vi "CCD_Exposure_2-D.vi"(7 "CCD GPIB Address":u16=1, 8 "error in":errorcluster, 10 "Shutter Enabled":bool=TRUE, 11 "Exposuretime (s)":dbl=0.5 format="%.2f") -> (0 "Error Out":errorcluster, 1 "#PixelOverflow":u32, 2 "PixelOverflow":bool, 3 "The Data":i32[][](array[numeric]), 4 "SD":i32=1024, 5 "1-D data":i32[](graph)=[177496, 177237, 176545, 175663, 175741, 175858, 175364, 175697, 175129, 174991, 175361, 175049, 173976, 174267, 174715, 174635, 174464, 174415, 174713, 174154, 174258, 174337, 173766, 174440, 174836, 174872, 175484, 175380, 175517, 175102, 176092, 175373, 177070, 176721, 176679, 176652, 176571, 177207, 176449, 176451, 176423, 175916, 176475, 176612, 176252, 176325, 176549, 176615, 176346, 176479, 175031, 175855, 175811, 175987, 175754, 176075, 175744, 176016, 176357, 176668, 175778, 176616, 176413, 176166, 176151, 176171, 176217, 176658, 176512, 175690, 176874, 176617, 176661, 176440, 176822, 176737, 176660, 176897, 177128, 176173, 176955, 177131, 176857, 177057, 177128, 177374, 177408, 177629, 176564, 177537, 178203, 177779, 177922, 178109, 178176, 177927, 177938, 178018, 178044, 178507, 178492, 178457, 178751, 178462, 179124, 178828, 178898, 178567, 179197, 179313, 179250, 178875, 179058, 179277, 179500, 179982, 179462, 179335, 179263, 179484, 179481, 179479, 179610, 179444, 179554, 179661, 178821, 179552, 179705, 179488, 179515, 179423, 179453, 179461, 179755, 179369, 179414, 179479, 179807, 179976, 179789, 179795, 179568, 179889, 179778, 178767, 179542, 179786, 179938, 179612, 179142, 179106, 179581, 179567, 178634, 178623, 179068, 178940, 178900, 178928, 179101, 178915, 178740, 178763, 177499, 178666, 178321, 178221, 178009, 178053, 177909, 177925, 177857, 177602, 177533, 177626, 177249, 177582, 177192, 176946, 177060, 176820, 176649, 175734, 176509, 176182, 176157, 176331, 176091, 176038, 175744, 176229, 175506, 175197, 175508, 175642, 175167, 175458, 175353, 175323, 175173, 175444, 174506, 175316, 175313, 175117, 174765, 174432, 175002, 174688, 174440, 173961, 174115, 174147, 174093, 173735, 173903, 173716, 173765, 173610, 173748, 173011, 173245, 173618, 173124, 173369, 173061, 173038, 172885, 172760, 172514, 172554, 173031, 173023, 172516, 172523, 172672, 172471, 172237, 172188, 171433, 171984, 171753, 171872, 171783, 171471, 171189, 171110, 171274, 170575, 171120, 171106, 171110, 170929, 171173, 170662, 170816, 170628, 170624, 170225, 170081, 170283, 170029, 169998, 169688, 169824, 169406, 169878, 169063, 169720, 169510, 169519, 169860, 169714, 169518, 169643, 169456, 169521, 168869, 169560, 168783, 168901, 168990, 169036, 168442, 168777, 168687, 168072, 168399, 168649, 168267, 168269, 168356, 168516, 168271, 168527, 167836, 167485, 167850, 167521, 167426, 167557, 167423, 167443, 167534, 167009, 166530, 167863, 167026, 166940, 167186, 166745, 166891, 166955, 166869, 167115, 165754, 166348, 166107, 166618, 166316, 166267, 166555, 166327, 166013, 165723, 166506, 166349, 165892, 166071, 166190, 165856, 165930, 165701, 165506, 164608, 165119, 165024, 165449, 165200, 165259, 165019, 165349, 164958, 164096, 165006, 164981, 164335, 164861, 164810, 164423, 164483, 164340, 164250, 163491, 164245, 164320, 163963, 163883, 163507, 163916, 164060, 164046, 162766, 163198, 163532, 163551, 163543, 162990, 163030, 163314, 163224, 162808, 162701, 162758, 162941, 163168, 162957, 163135, 162477, 162607, 162991, 161590, 162713, 162532, 162527, 162445, 162391, 162501, 162180, 162584, 162352, 162069, 162010, 161850, 162592, 162134, 161802, 161889, 161835, 162271, 161372, 161806, 161901, 161746, 161668, 161955, 161987, 161665, 161955, 161624, 161234, 161128, 161451, 161255, 161395, 161342, 161345, 161407, 161028, 160195, 161186, 160747, 160842, 160504, 160787, 160732, 160423, 160488, 160268, 159891, 159897, 160079, 160098, 160144, 159838, 160097, 160087, 159870, 159061, 159506, 159511, 159803, 159529, 159439, 159512, 158853, 159324, 158534, 159173, 159332, 158882, 159051, 158572, 158514, 158829, 158706, 158748, 157912, 158607, 158090, 158227, 158152, 158030, 158266, 158548, 158016, 157962, 158035, 157954, 157812, 157606, 157874, 157821, 157764, 157655, 157657, 156469, 156933, 156940, 156737, 156720, 156676, 156742, 156663, 156501, 156267, 156025, 156139, 156305, 155684, 155848, 155778, 156013, 155699, 155868, 155073, 155035, 154988, 155147, 155006, 154801, 154951, 154756, 154369, 154043, 154641, 154227, 154445, 154230, 154204, 154021, 153772, 153607, 154029, 152755, 153333, 153458, 153185, 152741, 152835, 152962, 152667, 152345, 151613, 152074, 152206, 152113, 151817, 151704, 151180, 151839, 151412, 150982, 150417, 151000, 150816, 150477, 150540, 150350, 150468, 150158, 149893, 149892, 149892, 149939, 149467, 149632, 149759, 149220, 148925, 149026, 148528, 147863, 148334, 148442, 148328, 147973, 148089, 148183, 148195, 147150, 146769, 147095, 147236, 146926, 146726, 146613, 146268, 146185, 145926, 146010, 144893, 145439, 145063, 145105, 144597, 144535, 143936, 143844, 143722, 142725, 142943, 143042, 142449, 142272, 142469, 141769, 141972, 141248, 141044, 140226, 140827, 140698, 140582, 139873, 140115, 139849, 139848, 139546, 138440, 138703, 138359, 138382, 138330, 137878, 137475, 137443, 137045, 136996, 136153, 136373, 136062, 135957, 135597, 135569, 135341, 135358, 135207, 133688, 134368, 133832, 134099, 133500, 133809, 133295, 132918, 132596, 131737, 131215, 131598, 130920, 131159, 130586, 129849, 130121, 129509, 129389, 128346, 128603, 127886, 127724, 127466, 127149, 126899, 126396, 126106, 125250, 125243, 125186, 124756, 124152, 124208, 123733, 123689, 123302, 122709, 121638, 122192, 121550, 121617, 121037, 121065, 121206, 120503, 120291, 120082, 119444, 119479, 119102, 119126, 118821, 119007, 119014, 118790, 118557, 117857, 118423, 117958, 118209, 118033, 117577, 117864, 117940, 117602, 117323, 117173, 117415, 117204, 117219, 116831, 117214, 116727, 116894, 116543, 116291, 116423, 116250, 116254, 115966, 115960, 116156, 115985, 115893, 115539, 115492, 115586, 115303, 115517, 115319, 115197, 115309, 114934, 115043, 114792, 114926, 114745, 114650, 114608, 114556, 114530, 114548, 114068, 113966, 114303, 114062, 114250, 113447, 113715, 113923, 113602, 113622, 113621, 113042, 113452, 113341, 113201, 113118, 113203, 112990, 112896, 112779, 112551, 112388, 112593, 112630, 112401, 112398, 112425, 112142, 112350, 112104, 111345, 111918, 111650, 111627, 111487, 111664, 111526, 111384, 111199, 111222, 111185, 111051, 111127, 110794, 110856, 111102, 110991, 110891, 110806, 110318, 110703, 110754, 110560, 110283, 110215, 110234, 110522, 110338, 109585, 110017, 109557, 109843, 109787, 109970, 109426, 109645, 109169, 109373, 108726, 109269, 109089, 109002, 109200, 109471, 108942, 109150, 108845, 108649, 108633, 108861, 108788, 108644, 108488, 108826, 108492, 108466, 108611, 107787, 107908, 108145, 108047, 107821, 107704, 107751, 107942, 107756, 107019, 107515, 107226, 107147, 107147, 107373, 107606, 106987, 107275, 106973, 106570, 106853, 107103, 106538, 106818, 106677, 106780, 106598, 106569, 106075, 106391, 106148, 106190, 106330, 106036, 106176, 106260, 106130, 105583, 105341, 105443, 105751, 105576, 105607, 105404, 105402, 105428, 105391, 104782, 105311, 105399, 105205, 104839, 105129, 105010, 104872, 104917, 104547, 104139, 104521, 104271, 104632, 104550, 104222, 104145, 104298, 104354, 103669, 104110, 103604, 104021, 103788, 103749, 103773, 103624, 103645, 103361, 103629, 103258, 103289, 103247, 103211, 103330, 103247, 103436, 103179, 102579, 102963, 102898, 102864, 102648, 102776, 102586, 102631, 102257, 102254, 102088, 102615, 102228, 102414, 102386, 102025, 101999, 101883, 101846, 101309, 101626, 101609, 101613, 101571, 101653, 101255, 101350, 101514, 100925, 100796, 101115, 100842, 101202, 100630, 100907, 100811, 100773, 100654, 100153, 100255, 100664, 100226, 100257, 100301, 99998, 100192, 99883, 99797, 99144, 99679, 99809, 99363, 99594, 99253, 99180, 99343, 99103, 98304, 99091, 98839, 98869, 98550, 98599, 98609, 98348, 98588, 98238, 97988, 98192, 97809, 97831, 97989, 97745, 97967, 97680, 97445, 96931, 97422, 97486, 97364, 97247, 97010, 96943, 96835, 96708, 96620, 96687, 96317, 96392, 96030, 96281, 95988, 96006, 95720, 96009, 95349, 95599, 95334, 95322, 95474, 95161, 95122, 94994, 95082, 94621, 94507, 94795, 94877, 94686, 94852, 94530, 94409, 94757, 94791, 94046, 94197, 94237, 94125, 93995, 94019, 94245, 94207, 94286, 93544, 93928, 93947, 93713, 94034, 93985, 91259], 6 "Setup String":string="ldb,1,0,u,0,180,30,b,1,76;sdu,0,1024,1024;cl0;omrt;sron;she;ex0.2")   [LabVIEW 2020]
doc: "Get the 2-D CCD data. The CCD GPIB address is more or less fixed.\nThe setup string uses global variable."
uses:
  Globals and TypeDefs/Type Definitions.llb/3 way Status.ctl
  Globals and TypeDefs/gStatus.vi
  Globals and TypeDefs/gDetector.vi
panel:
  out "SRQ":bool[](array[boolean])
  out "Trailing Byte":bool[](array[boolean])
  out "Trailing Byte Str":string
  out "#Mismatched":u32
  out "Bytes for Readout":i32
  out "Read String length":i32
  out "#Read Error":u32
  out "#SRQ Error":u32
  out "#Shots":u32
  out "Intensity Graph":i32[][](graph)
  out "Current State":T1(ring)=enum."Send Command"
  out "Data Dimensions":i32[](array[numeric])=[1024, 30]
  out "read":bool[](array[boolean])=[FALSE, FALSE, FALSE, FALSE, FALSE, FALSE, FALSE, FALSE, TRUE, FALSE, FALSE, FALSE, FALSE, TRUE, FALSE, FALSE]
  out "TS":bool[](array[boolean])
  out "ST":bool[](array[boolean])=[FALSE, FALSE, FALSE, FALSE, FALSE, FALSE, FALSE, FALSE, TRUE, FALSE, FALSE, FALSE, FALSE, FALSE, FALSE, FALSE]
  out "SRQ poll response":i16=65
  out "InitialArray Length":i32=30720
  out "LD":i32=30
  # "Acc overflow"
  # "FIFO overflow"
  # "Exp halted by user"
  # "Status Byte:\n[0]: Dev.Clear State  \n[1]: Dev.Trig.State    \n[2]: Listener Active   \n[3]: Talker Active      \n[4]: Attn. Asserted    \n[5]: CIC                      \n[6]: Remote State       \n[7]: Lockout State      \n[8]: Oper.Complete\n[9]:   ---\n[10]: ---\n[11]: ---\n[12]: SRQ det.whl CIC\n[13]: EOI or EOS det.\n[14]: Timeout\n[15]: Error detected"
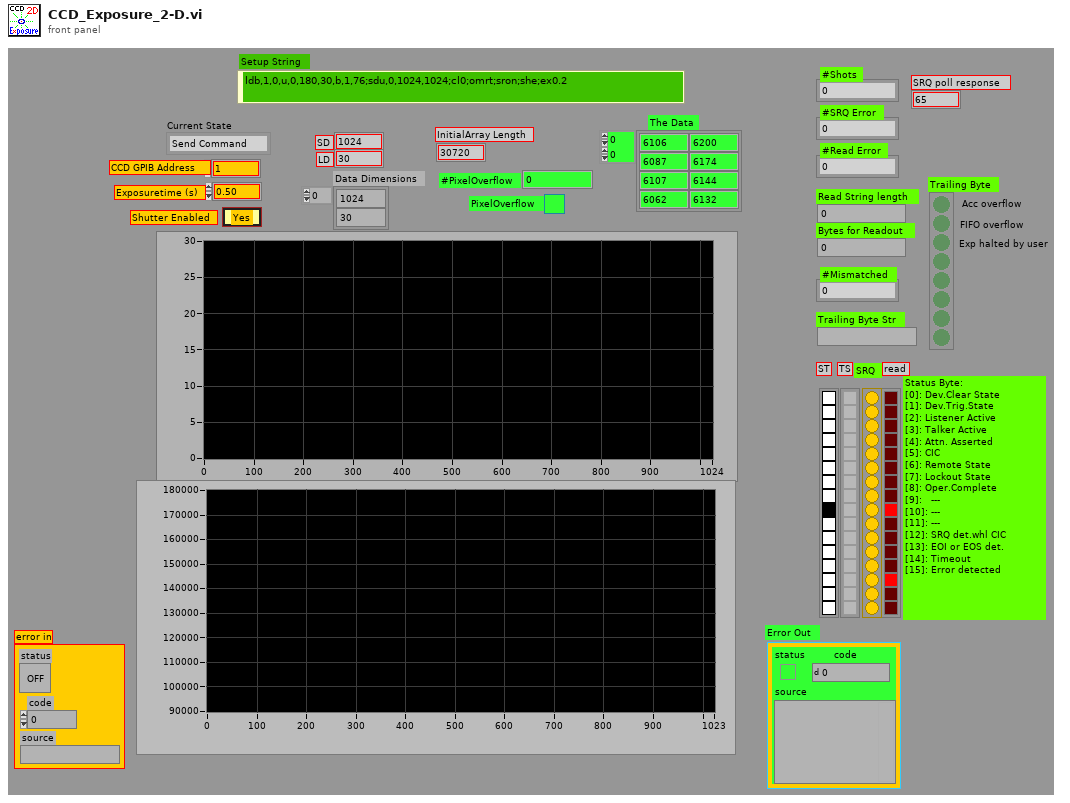
[diagram p1: front panel]
types:
  T1 = enum16{"__Quit__", "Send Command", "Wait", "Check SRQ", "Receive Data"}
  T2 = typedef "3 way Status.ctl" = u8
  T3 = enum16{"__Quit__", "Send Command", "Wait", "Check SRQ", "Receive Data", "Process Data"}
  T4 = enum16{"--Quit--", "Init GPIB", "Poll GPIB", "Wait for SRQ", "Clear CCD Parameters", "New CCD Parameters", "Check CCD Command Error"}
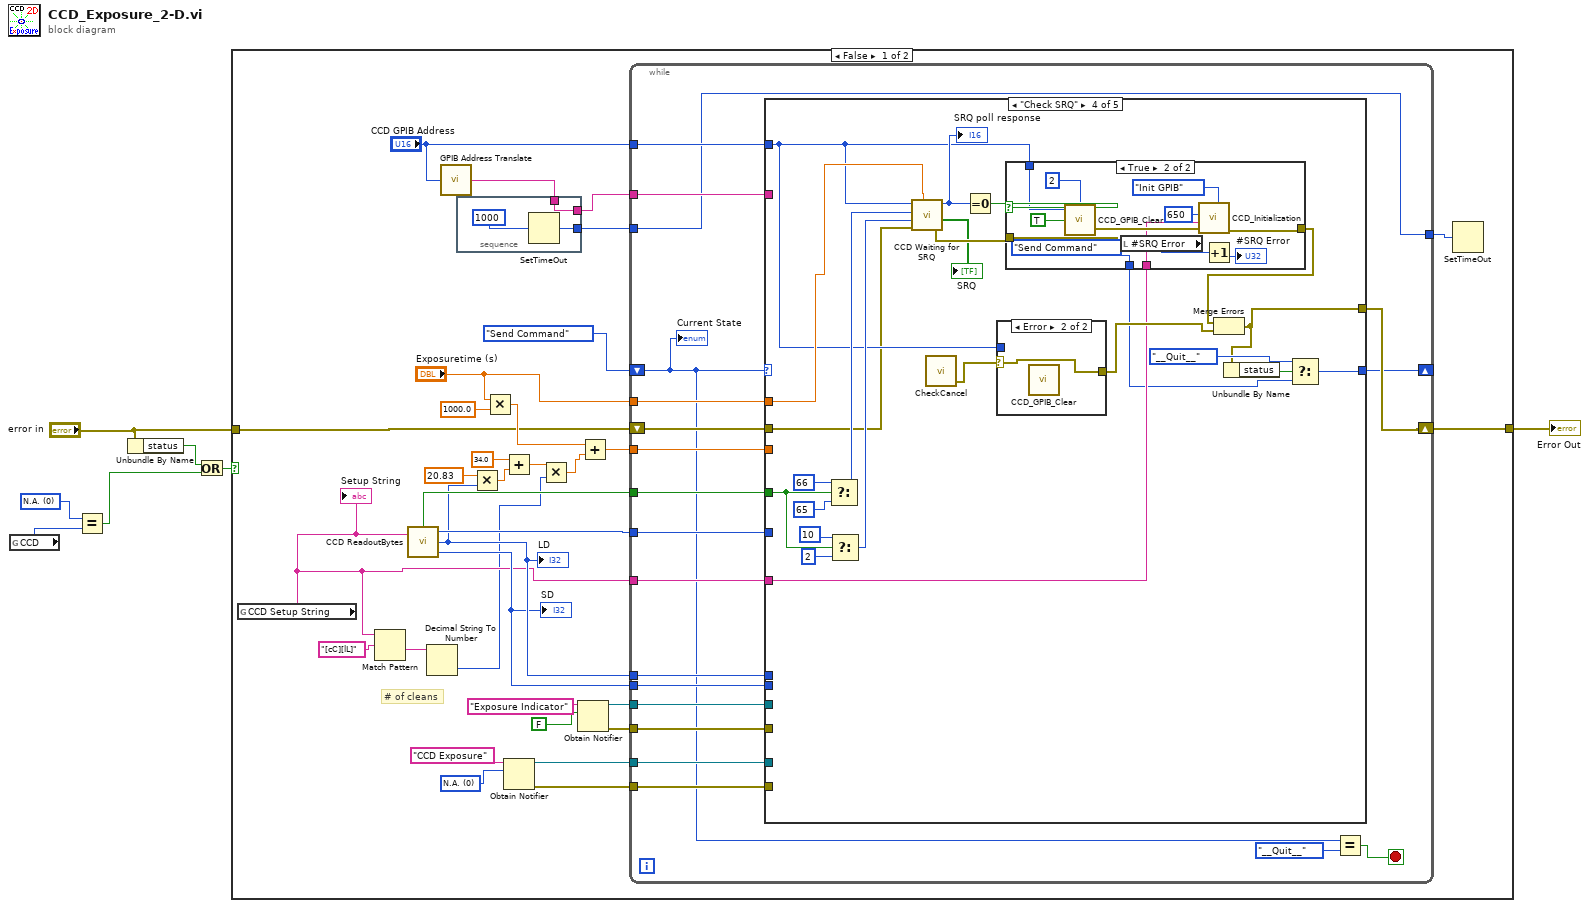
[diagram p0: block diagram]
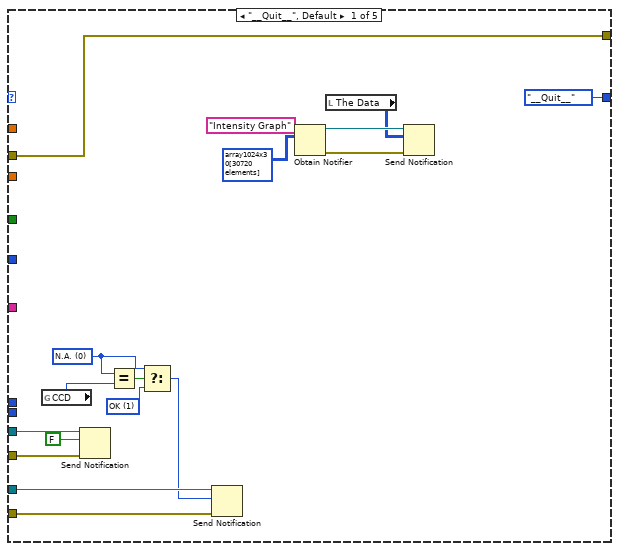
[diagram p2: hidden frame]
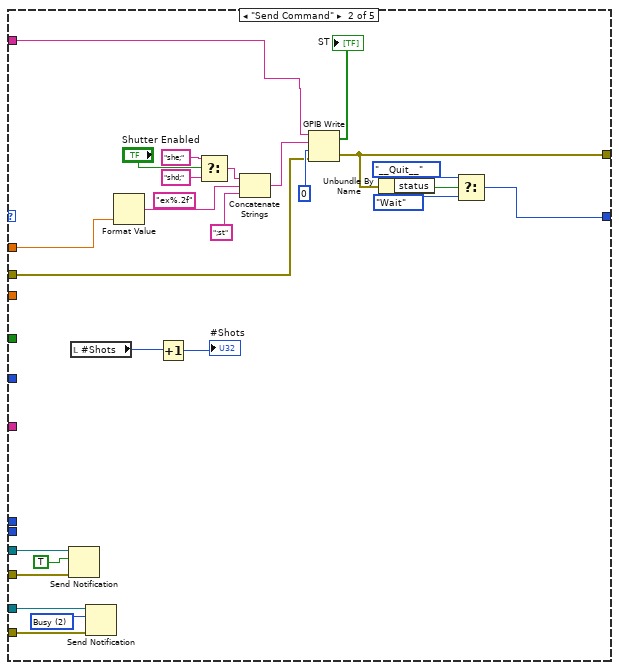
[diagram p3: hidden frame]
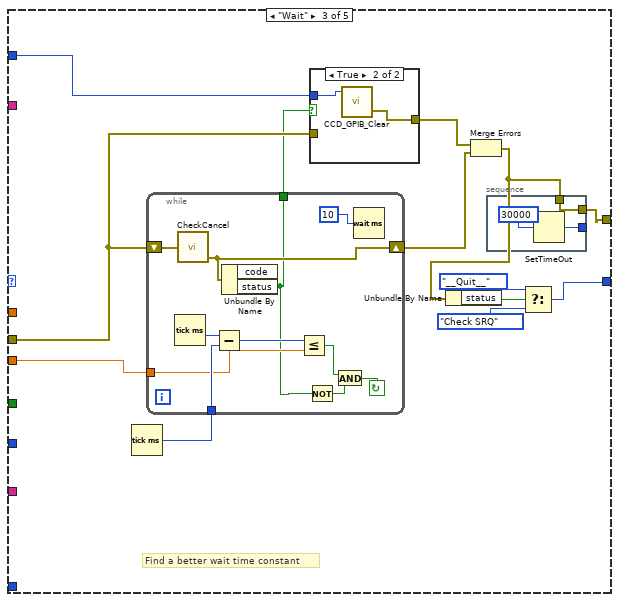
[diagram p4: hidden frame]
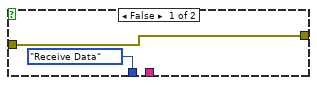
[diagram p6: hidden frame]
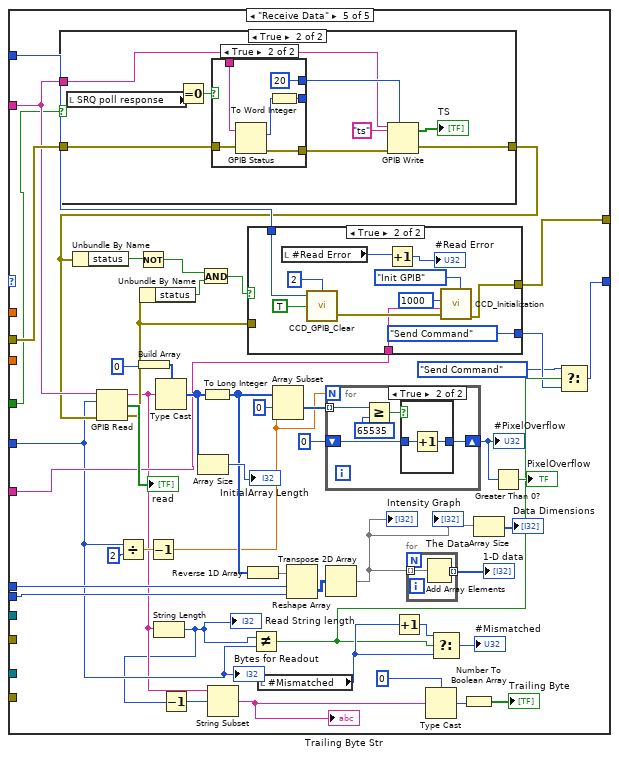
[diagram p8: hidden frame]
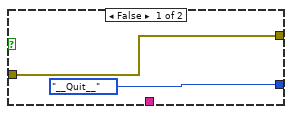
[diagram p9: hidden frame]
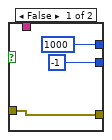
[diagram p11: hidden frame]
diagram:
  w5 = T2 0 items=["N.A.", "OK", "Busy", "Done"] ("y")
  n1 = global read "gStatus.vi" "CCD"() -> (w6:T2)
  n2 = Equal?(x=w5, y=w6) -> (x = y?=w3:bool)
  n3 = Unbundle By Name("error in") -> ("status"=w2:bool)
  n4 = Or(x=w2, y=w3) -> (x .or. y?=w4:bool)
  n5 = case shown="False" w4 {
    tunnel: [w27 w265] -> w7
    tunnel: "error in" -> [w25 w265]
    frame False {
      w14 = T2 0 items=["N.A.", "OK", "Busy", "Done"] ("Saving")
      # "# of cleans"
      n6 = global read "gDetector.vi" "CCD Setup String"() -> (w20:string)
      "Setup String" <- w20
      n7 = Match Pattern(string=w20, regular expression="[cC][lL]") -> (after substring=w21:string)  [unwired: 1 in, 3 out]
      n8 = call "CCD ReadoutBytes.vi"("CCD Setup String"=w20) -> ("RM(T) or RT(F) mode"=w37:bool, "Bytes for Readout"=w38:i32, "LD Bytes"=w29:i32, "SD Bytes"=w28:i32)  [unwired: 1 in]
      "SD" <- w28
      "LD" <- w29
      n9 = Decimal String To Number(string=w21) -> (number=w18:i32)  [unwired: 2 in, 1 out]
      n10 = call "GPIB Address Translate.vi"("GPIB Address"="CCD GPIB Address") -> ("GPIB Address String"=w40:string)
      n11 = stacked-sequence {
        tunnel: [w42] -> w39
        tunnel: w40 -> [w42]
        tunnel: [w41] -> w24
        frame #0 {
          n12 = SetTimeOut(1:1000) -> (0:w41:i32)
        }
      }
      n13 = Multiply(x=20.83, y=w29) -> (x*y=w35:dbl)
      n14 = Multiply(x="Exposuretime (s)", y=1000.0) -> (x*y=w31:dbl)
      n15 = Add(x=34.0, y=w35) -> (x+y=w19:dbl)
      n16 = Obtain Notifier(name (unnamed)="CCD Exposure", notification data type=w14) -> (notifier out=w13:refnum<notifier>, error out=w12:errorcluster)  [unwired: 2 in, 1 out]
      n17 = Multiply(x=w19, y=w18) -> (x*y=w17:dbl)
      n18 = Obtain Notifier(name (unnamed)="Exposure Indicator", notification data type=FALSE ("SaveData?")) -> (notifier out=w9:refnum<notifier>, error out=w8:errorcluster)  [unwired: 2 in, 1 out]
      n19 = Add(x=w31, y=w17) -> (x+y=w16:dbl)
      n20 = while {
        shift-right: [w59] -> _
        shift-left: T1."Send Command" ("Starting Mode") -> [w44]
        tunnel: w39 -> [w63]
        shift-right: [w61] -> w27
        shift-left: w25 -> [w62]
        tunnel: w38 -> [w56]
        tunnel: w37 -> [w57]
        tunnel: "Exposuretime (s)" -> [w60]
        tunnel: "CCD GPIB Address" -> [w58]
        tunnel: w29 -> [w55]
        tunnel: w28 -> [w54]
        tunnel: w20 -> [w51]
        tunnel: w24 -> [w50]
        tunnel: [w50] -> w23
        tunnel: w16 -> [w49]
        tunnel: w13 -> [w48]
        tunnel: w12 -> [w47]
        tunnel: w9 -> [w46]
        tunnel: w8 -> [w45]
        stop <- w53 stop-if-true
        n21 = case shown="\"Check SRQ\"" w44 {
          tunnel: w63 -> [_ w96 _ _ w204]
          tunnel: w62 -> [w77 w95 w115 w138 w222]
          tunnel: [w77 w93 w108 w154 w191] -> w61
          tunnel: w60 -> [_ w94 _ w147 _]
          tunnel: [T3."__Quit__" w89 w111 w153 w177] -> w59
          tunnel: w58 -> [_ _ w118 w140 w198]
          tunnel: w57 -> [_ _ _ w151 w199]
          tunnel: w56 -> [_ _ _ _ w189]
          tunnel: w55 -> [_ _ _ _ w203]
          tunnel: w54 -> [_ _ _ _ w202]
          tunnel: w51 -> [_ _ _ w142 w190]
          tunnel: w49 -> [_ _ w110 _ _]
          tunnel: w48 -> [w79 w86 _ _ _]
          tunnel: w47 -> [w78 w85 _ _ _]
          tunnel: w46 -> [w71 w83 _ _ _]
          tunnel: w45 -> [w70 w82 _ _ _]
          frame "__Quit__", Default {
            w73 = T2 1 items=["N.A.", "OK", "Busy", "Done"] ("f")
            w74 = T2 0 items=["N.A.", "OK", "Busy", "Done"] ("y")
            n22 = global read "gStatus.vi" "CCD"() -> (w75:T2)
            n23 = Send Notification(notification=FALSE, notifier=w71, error in (no error)=w70) -> ()  [unwired: 2 out]
            n24 = Equal?(x=w74, y=w75) -> (x = y?=w76:bool)
            n25 = Select(t=w74, s=w76, f=w73) -> (s? t:f=w72:T2)
            n26 = Send Notification(notification=w72, notifier=w79, error in (no error)=w78) -> ()  [unwired: 2 out]
            n27 = Obtain Notifier(name (unnamed)="Intensity Graph", notification data type=i32[][] array1024x30[30720 elements] ("Intensity Graph")) -> (notifier out=w66:refnum<notifier>, error out=w65:errorcluster)  [unwired: 2 in, 1 out]
            n28 = local read "The Data"() -> (w64:i32[][])
            n29 = Send Notification(notification=w64, notifier=w66, error in (no error)=w65) -> ()  [unwired: 2 out]
          }
          frame "Send Command" {
            w84 = T2 2 items=["N.A.", "OK", "Busy", "Done"] ("notification")
            n30 = Send Notification(notification=TRUE, notifier=w83, error in (no error)=w82) -> ()  [unwired: 2 out]
            n31 = local read "#Shots"() -> (w87:u32)
            n32 = Send Notification(notification=w84, notifier=w86, error in (no error)=w85) -> ()  [unwired: 2 out]
            n33 = Format Value(format string="ex%.2f", value (0)=w94) -> (output string=w104:string)  [unwired: 1 in]
            n34 = Increment(x=w87) -> (x+1=→"#Shots":u32)
            n35 = Select(t="she;", s="Shutter Enabled", f="shd;") -> (s? t:f=w103:string)
            n36 = Concatenate Strings(w103, w104, ";st") -> (w105:string)
            n37 = GPIB Write(0:w96, 1:w105, 2:i16 0 ("mode (0)"), 3:w95) -> (5:→"ST":bool[], 6:w93:errorcluster)  [unwired: 1 in]
            n38 = Unbundle By Name(w93) -> ("status"=w92:bool)
            n39 = Select(t=T3."__Quit__", s=w92, f=T3."Wait" ("Starting Mode")) -> (s? t:f=w89:T3)
          }
          frame "Wait" {
            # "Find a better wait time constant"
            n40 = Tick Count (ms)() -> (millisecond timer value=w119:u32)
            n41 = while {
              tunnel: w110 -> [w133]
              tunnel: w119 -> [w135]
              shift-right: [w127] -> w116
              shift-left: w115 -> [w128]
              tunnel: [w126] -> w109
              stop <- w130 continue-if-true
              n42 = Tick Count (ms)() -> (millisecond timer value=w136:u32)
              n43 = call "CheckCancel.vi"("error in (no error)"=w128) -> ("error out"=w127:errorcluster)  [unwired: 1 in, 1 out]
              n44 = Subtract(x=w136, y=w135) -> (x-y=w129:u32)
              n45 = Unbundle By Name(w127) -> ("status"=w126:bool)  [unwired: 1 out]
              n46 = Less Or Equal?(x=w129, y=w133) -> (x <= y?=w131:bool)
              n47 = Not(x=w126) -> (.not. x?=w132:bool)
              n48 = And(x=w131, y=w132) -> (x .and. y?=w130:bool)
              n49 = Wait (ms)(milliseconds to wait=u32 10 ("millisecond multiple")) -> ()  [unwired: 1 out]
            }
            n50 = case shown="True" w109 {
              tunnel: w118 -> [_ w124]
              tunnel: [w123 w125] -> w117
              tunnel: w115 -> [w123 _]
              frame False {
              }
              frame True {
                n51 = call "CCD_GPIB_Clear.vi"("GPIB Address"=w124) -> ("error out"=w125:errorcluster)  [unwired: 4 in]
              }
            }
            n52 = Merge Errors(w117, w116) -> (w107:errorcluster)
            n53 = Unbundle By Name(w107) -> ("status"=w114:bool)
            n54 = stacked-sequence {
              tunnel: [w121] -> w108
              tunnel: w107 -> [w121]
              tunnel: [w120] -> _
              frame #0 {
                n55 = SetTimeOut(1:30000) -> (0:w120:i32)
              }
            }
            n56 = Select(t=T3."__Quit__", s=w114, f=T3."Check SRQ" ("Starting Mode")) -> (s? t:f=w111:T3)
          }
          frame "Check SRQ" {
            n57 = Select(t=i16 66, s=w151, f=i16 65 ("y")) -> (s? t:f=w157:i16)
            n58 = Select(t=i16 10, s=w151, f=i16 2) -> (s? t:f=w148:i16)
            n59 = call "CCD Waiting for SRQ.vi"("Exposuretime (s)"=w147, "error in"=w138, "time loop constant"=w148, "poll status waiting for"=w157, "GPIB Address"=w140) -> ("error out"=w143:errorcluster, "Poll Status"=→"SRQ":bool[], "Poll Byte"=w146:i16)  [unwired: 1 out]
            "SRQ poll response" <- w146
            n60 = call "CheckCancel.vi"() -> ("error out"=w137:errorcluster)  [unwired: 2 in, 1 out]
            n61 = Equal To 0?(x=w146) -> (x = 0?=w145:bool)
            n62 = case shown="Error" w137 {
              selector: w137 -> [w173 w174]
              tunnel: w140 -> [_ _]
              tunnel: [w173 w174] -> w152
              frame No Error {
              }
              frame Error {
                n63 = call "CCD_GPIB_Clear.vi"() -> ()  [unwired: 5 in, 1 out]
              }
            }
            n64 = case shown="True" w145 {
              tunnel: w140 -> [_ w172]
              tunnel: [w161 w168] -> w144
              tunnel: w143 -> [w161 _]
              tunnel: w142 -> [_ w167]
              tunnel: [T3."Receive Data" ("Starting Mode") T3."Send Command" ("Starting Mode")] -> w141
              frame False {
              }
              frame True {
                n65 = call "CCD_GPIB_Clear.vi"("#device clearings"=2 ("#cleans"), "Device Clear?"=TRUE, "GPIB Address"=w172) -> ("error out"=w169:errorcluster)  [unwired: 2 in]
                n66 = local read "#SRQ Error"() -> (w162:u32)
                n67 = call "CCD_Initialization.vi"("milliseconds to wait"=u32 650, "Setup String"=w167, "error in"=w169, "Starting Action"=T4."Init GPIB") -> ("error out"=w168:errorcluster)  [unwired: 1 in, 4 out]
                n68 = Increment(x=w162) -> (x+1=→"#SRQ Error":u32)
              }
            }
            n69 = Merge Errors(w144, w152) -> (w154:errorcluster)
            n70 = Unbundle By Name(w154) -> ("status"=w156:bool)
            n71 = Select(t=T3."__Quit__", s=w156, f=w141) -> (s? t:f=w153:T3)
          }
          frame "Receive Data" {
            n72 = case shown="True" w199 {
              tunnel: w222 -> [w236 w241]
              tunnel: [w236 w240] -> w197
              tunnel: w204 -> [_ w239]
              frame False {
              }
              frame True {
                n73 = local read "SRQ poll response"() -> (w242:i16)
                n74 = Equal To 0?(x=w242) -> (x = 0?=w243:bool)
                n75 = case shown="True" w243 {
                  tunnel: w239 -> [_ w254]
                  tunnel: [i16 -1 w253] -> _
                  tunnel: [u32 1000 u32 20] -> w244
                  tunnel: w241 -> [w246 w250]
                  tunnel: [w246 w249] -> w245
                  frame False {
                  }
                  frame True {
                    n76 = GPIB Status(0:w254, 1:w250) -> (3:w252:i16, 5:w249:errorcluster)  [unwired: 2 out]
                    n77 = To Word Integer(number=w252) -> (16bit integer=w253:i16)
                  }
                }
                n78 = GPIB Write(0:w239, 1:"ts" ("String to Write"), 3:w245, 4:w244) -> (5:→"TS":bool[], 6:w240:errorcluster)  [unwired: 1 in]
              }
            }
            n79 = Unbundle By Name(w197) -> ("status"=w196:bool)
            n80 = GPIB Read(0:w204, 1:w189, 3:w197) -> (5:w185:string, 6:→"read":bool[], 7:w192:errorcluster)  [unwired: 2 in]
            n81 = Divide(x=w189, y=2) -> (x/y=w212:dbl)
            n82 = Not(x=w196) -> (.not. x?=w194:bool)
            n83 = Build Array(u16 0) -> (w219:u16[])
            n84 = Unbundle By Name(w192) -> ("status"=w195:bool)
            n85 = Decrement(x=w212) -> (x-1=w205:dbl)
            n86 = String Length(string=w185) -> (length=w183:i32)
            "Read String length" <- w183
            n87 = Type Cast(type=w219, x=w185) -> (*(type *) &x=w221:u16[])
            n88 = Decrement(x=w183) -> (x-1=w184:i32)
            n89 = Array Size(array=w221) -> (size(s)=→"InitialArray Length":i32)
            n90 = And(x=w194, y=w195) -> (x .and. y?=w193:bool)
            n91 = To Long Integer(number=w221) -> (32bit integer=w214:i32[])
            n92 = String Subset(string=w185, offset (0)=w184) -> (substring=w182:string)  [unwired: 1 in]
            "Trailing Byte Str" <- w182
            n93 = case shown="True" w193 {
              tunnel: w198 -> [_ w235]
              tunnel: [w224 w231] -> w191
              tunnel: w192 -> [w224 _]
              tunnel: w190 -> [_ w230]
              tunnel: [T3."__Quit__" ("Starting Mode") T3."Send Command" ("Starting Mode")] -> w176
              frame False {
              }
              frame True {
                n94 = local read "#Read Error"() -> (w225:u32)
                n95 = call "CCD_GPIB_Clear.vi"("#device clearings"=2 ("#cleans"), "Device Clear?"=TRUE, "GPIB Address"=w235) -> ("error out"=w232:errorcluster)  [unwired: 2 in]
                n96 = Increment(x=w225) -> (x+1=→"#Read Error":u32)
                n97 = call "CCD_Initialization.vi"("milliseconds to wait"=u32 1000, "Setup String"=w230, "error in"=w232, "Starting Action"=T4."Init GPIB") -> ("error out"=w231:errorcluster)  [unwired: 1 in, 4 out]
              }
            }
            n98 = Reverse 1D Array(array=w214) -> (reversed array=w216:i32[])
            n99 = Not Equal?(x=w183, y=w189) -> (x != y?=w178:bool)
            n100 = local read "#Mismatched"() -> (w186:u32)
            n101 = Array Subset(array=w214, index=0, length=w205) -> (w210:i32[])
            n102 = Reshape Array(w216, w203, w202) -> (w217:i32[][])
            n103 = for {
              N: w205 -> [_]
              tunnel: w210 -> [w260] mode=indexing
              shift-right: [w258] -> w208
              shift-left: u32 0 -> [w257]
              n104 = Greater Or Equal?(x=w260, y=65535) -> (x >= y?=w259:bool)
              n105 = case shown="True" w259 {
                tunnel: [w262 w264] -> w258
                tunnel: w257 -> [w262 w263]
                frame False {
                }
                frame True {
                  n106 = Increment(x=w263) -> (x+1=w264:u32)
                }
              }
            }
            "#PixelOverflow" <- w208
            n107 = Transpose 2D Array(2D array=w217) -> (transposed array=w200:i32[][])
            "The Data" <- w200
            "Intensity Graph" <- w200
            n108 = Increment(x=w186) -> (x+1=w188:u32)
            n109 = for {
              tunnel: [w256] -> w201 mode=indexing
              tunnel: w200 -> [w255] mode=indexing
              n110 = Add Array Elements(numeric array=w255) -> (sum=w256:i32)
            }
            "1-D data" <- w201
            n111 = Type Cast(type=u8 0, x=w182) -> (*(type *) &x=w180:u8)
            n112 = Select(t=w188, s=w178, f=w186) -> (s? t:f=→"#Mismatched":u32)
            n113 = Number To Boolean Array(number=w180) -> (Boolean array=→"Trailing Byte":bool[])
            n114 = Array Size(array=w200) -> (size(s)=→"Data Dimensions":i32[])
            n115 = Greater Than 0?(x=w208) -> (x > 0?=→"PixelOverflow":bool)
            n116 = Select(t=T3."Send Command" ("Starting Mode"), s=w178, f=w176) -> (s? t:f=w177:T3)
            "Bytes for Readout" <- w189
          }
        }
        n117 = Equal?(x=w44, y=T3."__Quit__") -> (x = y?=w53:bool)
        "Current State" <- w44
      }
      n118 = SetTimeOut(1:w23) -> ()  [unwired: 1 out]
    }
    frame True {
    }
  }
  "Error Out" <- w7
